vi "Initialize Camera and CheckList.vi"(11 "ListBox in":refnum<vi>) -> (1 "Cluster":cluster{"value":i32, "value":i32, "index":i32}, 2 "Array":cluster{string[]}[](array[cluster]), 3 "File Refnum":T1)   [LabVIEW 2013]
uses:
  <vilib>/Utility/config.llb/Config Data RefNum.ctl
  <vilib>/Utility/config.llb/Read Key (String).vi
  <vilib>/Utility/config.llb/Read Key (I32).vi
  <vilib>/Utility/config.llb/NI_LVConfig.lvlib
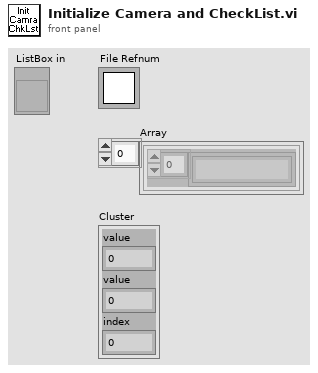
[diagram p1: front panel]
types:
  T1 = typedef "NI_LVConfig.lvlib/Config Data RefNum.ctl" = refnum<k1>
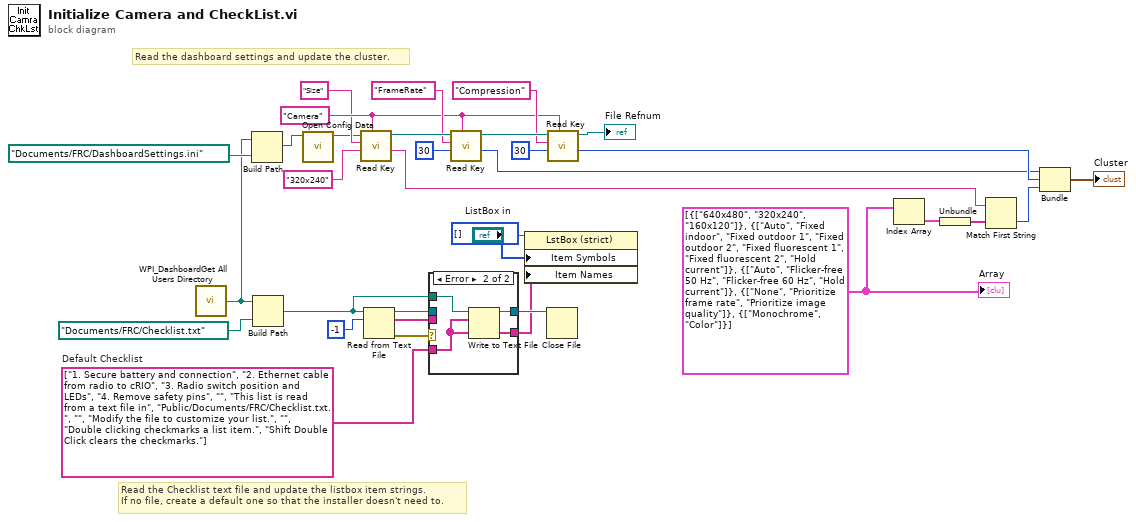
[diagram p0: block diagram]
diagram:
  w15 = "Camera"
  w23 = cluster{string[]}[] [{["640x480", "320x240", "160x120"]}, {["Auto", "Fixed indoor", "Fixed outdoor 1", "Fixed outdoor 2", "Fixed fluorescent 1", "Fixed fluorescent 2", "Hold current"]}, {["Auto", "Flicker-free 50 Hz", "Flicker-free 60 Hz", "Hold current"]}, {["None", "Prioritize frame rate", "Prioritize image quality"]}, {["Monochrome", "Color"]}]
  w8 = string[] ["1. Secure battery and connection", "2. Ethernet cable from radio to cRIO", "3. Radio switch position and LEDs", "4. Remove safety pins", "", "This list is read from a text file in", "Public/Documents/FRC/Checklist.txt.", "", "Modify the file to customize your list.", "", "Double clicking checkmarks a list item.", "Shift Double Click clears the checkmarks."]  # Default Checklist
  # "Read the Checklist text file and update the listbox item strings.\nIf no file, create a default one so that the installer doesn't need to."
  # "Read the dashboard settings and update the cluster."
  n1 = call <vilib>:"WPI_DashboardGet All Users Directory.vi"() -> ("All User Path"=w10:path)
  n2 = Build Path(base path=w10, name or relative path=path "Documents/FRC/DashboardSettings.ini") -> (appended path=w11:path)
  n3 = Build Path(base path=w10, name or relative path=path "Documents/FRC/Checklist.txt") -> (appended path=w7:path)
  n4 = call <vilib>:"Open Config Data.vi"("configuration file path"=w11) -> ("refnum"=w12:T1)  [unwired: 8 in, 2 out]
  n5 = call-poly <vilib>:"Read Key.vi"("section"=w15, "default value"="320x240", "key"="Size", "refnum"=w12) -> ("value"=w25:string, "refnum out"=w30:T1)  [unwired: 2 in, 4 out]
  n6 = Read from Text File(file (use dialog)=w7, count=-1 ("timeout ms (25000)")) -> (refnum out=w28:refnum<file>, text=w6:string[], error out=w5:errorcluster)  [unwired: 2 in, 1 out]
  n7 = case shown="Error" w5 {
    tunnel: w6 -> [w35 _]
    tunnel: [w35 w37] -> w9
    tunnel: w8 -> [_ w37]
    tunnel: w7 -> [_ w38]
    tunnel: [w34 w36] -> w29
    tunnel: w28 -> [w34 _]
    frame No Error {
    }
    frame Error {
      n8 = Write to Text File(file (use dialog)=w38, text=w37) -> (refnum out=w36:refnum<file>)  [unwired: 2 in, 2 out]
    }
  }
  n9 = call-poly <vilib>:"Read Key.vi"("section"=w15, "default value"=30, "key"="FrameRate", "refnum"=w30) -> ("value"=w20:i32, "refnum out"=w31:T1)  [unwired: 1 in, 5 out]
  n10 = property on="Property Node" class="LstBox (strict)"(reference="ListBox in", "Item Symbols"=i32[] [], "Item Names"=w9) -> ()  [unwired: 1 in, 2 out]
  n11 = Close File(refnum=w29) -> ()  [unwired: 1 in, 2 out]
  n12 = call-poly <vilib>:"Read Key.vi"("section"=w15, "default value"=30, "key"="Compression", "refnum"=w31) -> ("value"=w21:i32, "refnum out"=→"File Refnum":T1)  [unwired: 1 in, 5 out]
  n13 = Index Array(array=w23) -> (element=w22:cluster{string[]})  [unwired: 1 in]
  n14 = Unbundle(w22) -> (w24:string[])
  n15 = Match First String(2:w24, 3:w25) -> (0:w26:i32)  [unwired: 1 out]
  n16 = Bundle("value"=w20, "value"=w21, "index"=w26) -> (→"Cluster":cluster{"value":i32, "value":i32, "index":i32})  [unwired: 1 out]
  "Array" <- w23
